vi "SubVI_MultipleRead.vi"(8 "error in":errorcluster, 11 "String":string) -> (0 "error out":errorcluster, 2 "Data":variant[](array[variant]), 3 "Read status?":bool[](array[boolean]))   [LabVIEW 2022 SP3, in "ADS_Library.lvlib"]
doc: "Multiple TwinCAT value read, this VI creates a connection to many TwinCAT parameters.\nEach parameter is read once and cast to LV types, the handle is then released and data \npassed out in an array of variants."
uses:
  ADS_Library.lvlib
  <userlib>/Beckhoff-LabVIEW-Interface/_DependsOn/Base/Read/Read Sync.vi
  <userlib>/Beckhoff-LabVIEW-Interface/_DependsOn/Base/TypeResolver/Get TypeResolver.vi
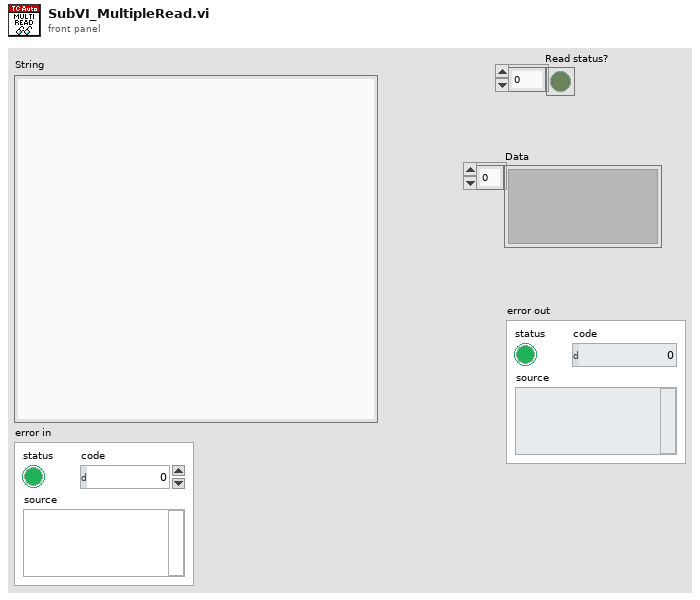
[diagram p1: front panel]
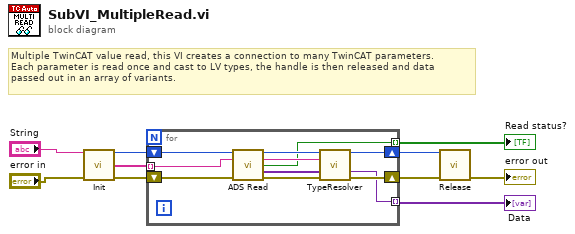
[diagram p0: block diagram]
diagram:
  # "Multiple TwinCAT value read, this VI creates a connection to many TwinCAT parameters.\nEach parameter is read once and cast to LV types, the handle is then released and data \npassed out in an array of variants."
  n1 = call <userlib>:"Init.vi"("XMLDescription"="String", "error in (no error)"="error in") -> ("Handle"=w8:u32, "ReadGrpSymbols"=w7:string[], "error out"=w9:errorcluster)  [unwired: 9 in, 2 out]
  n2 = for {
    tunnel: w7 -> [w11] mode=indexing
    tunnel: [w13] -> w3 mode=indexing
    tunnel: [w12] -> w2 mode=indexing
    shift-right: [w15] -> w6
    shift-left: w9 -> [w21]
    shift-right: [w14] -> w5
    shift-left: w8 -> [w20]
    n3 = call-poly <userlib>:"ADS Read.vi"("Handle"=w20, "SymbolName"=w11, "error in (no error)"=w21) -> ("Handle"=w19:u32, "SymbolName"=w18:string, "Read status?"=w13:bool, "Ads Read Data"=w17:variant[], "error out"=w16:errorcluster)  [unwired: 8 in]
    n4 = call-poly <userlib>:"TypeResolver.vi"("Handle"=w19, "SymbolName"=w18, "ADSRData"=w17, "error in"=w16) -> ("Handle"=w14:u32, "RData"=w12:variant, "error out"=w15:errorcluster)  [unwired: 8 in, 1 out]
  }
  "Read status?" <- w3
  "Data" <- w2
  n5 = call <userlib>:"Release.vi"("Handle"=w5, "error in (no error)"=w6) -> ("error out"=→"error out":errorcluster)  [unwired: 13 in]
